vi "Keithley 230 Voltage Ramp.vi"(2 "Point #":i32, 4 "Parameters":dbl[](array[numeric])=[0.0, 1e-09, 1e-08] format="%.3e", 5 "Instrument Address":refnum<visa-resource-name>) -> (0 "Stop":bool, 1 "Keithley 230 Voltage":dbl[](array[numeric]) format="%.2e")   [LabVIEW 2020]
panel:
  # "Start V"
  # "Increment V"
  # "Stop V"
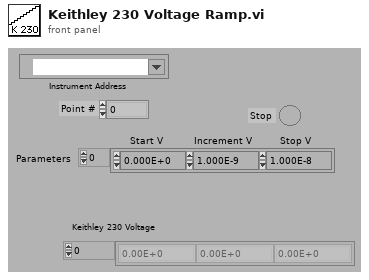
[diagram p1: front panel]
types:
  T1 = cluster{"Parameters[0]":dbl, "Parameters[1]":dbl, "Parameters[2]":dbl}
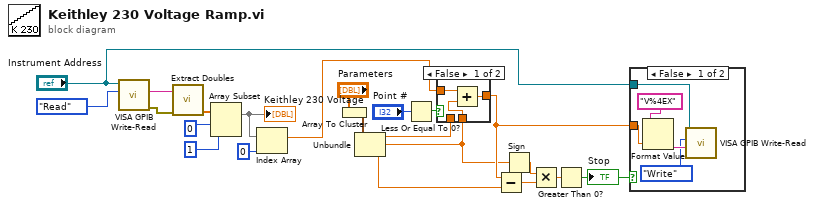
[diagram p0: block diagram]
diagram:
  n1 = call "VISA GPIB Write-Read.vi"("Action"=enum16{"Write", "Read", "Write & Read"}."Read", "VISA resource name"="Instrument Address") -> ("error out"=w1:errorcluster, "String Returned"=w6:string)  [unwired: 6 in, 2 out]
  n2 = call "Extract Doubles.vi"("error in"=w1, "String"=w6) -> ("Data"=w7:dbl[])  [unwired: 4 in, 1 out]
  n3 = Array Subset(array=w7, index=0, length=1) -> (w4:dbl[])
  "Keithley 230 Voltage" <- w4
  n4 = Index Array(array=w4, index=0) -> (element=w5:dbl)
  n5 = Array To Cluster(array="Parameters") -> (cluster=w11:T1)
  n6 = Unbundle(w11) -> ("Parameters[0]"=w21:dbl, "Parameters[1]"=w20:dbl, "Parameters[2]"=w13:dbl)
  n7 = Less Or Equal To 0?(x="Point #") -> (x <= 0?=w18:bool)
  n8 = case shown="False" w18 {
    tunnel: [w24 w26] -> w22
    tunnel: w21 -> [_ w26]
    tunnel: w5 -> [w25 _]
    tunnel: w20 -> [w23 _]
    frame False {
      n9 = Add(x=w25, y=w23) -> (x+y=w24:dbl)
    }
    frame True {
    }
  }
  n10 = Subtract(x=w22, y=w13) -> (x-y=w15:dbl)
  n11 = Sign(1:w20) -> (0:w17:dbl)
  n12 = Multiply(x=w17, y=w15) -> (x*y=w16:dbl)
  n13 = Greater Than 0?(x=w16) -> (x > 0?=w14:bool)
  "Stop" <- w14
  n14 = case shown="False" w14 {
    tunnel: "Instrument Address" -> [w29 _]
    tunnel: w22 -> [w30 _]
    frame False {
      n15 = Format Value(format string="V%4EX", value (0)=w30) -> (output string=w28:string)  [unwired: 1 in]
      n16 = call "VISA GPIB Write-Read.vi"("Command"=w28, "Action"=enum16{"Write", "Read", "Write & Read"}."Write", "VISA resource name"=w29) -> ()  [unwired: 5 in, 4 out]
    }
    frame True {
    }
  }
